vi "Laplacian_kernel.vi"(8 "error in":errorcluster caption="entrée d'erreur", 9 "Y":string[][](array[string]), 10 "X":string[][](array[string]), 11 "laplacian_kernel":cluster{"gamma":string}={"gamma"="None"}) -> (0 "error out":errorcluster caption="sortie d'erreur", 3 "Data":T1)   [LabVIEW 2020]
doc: "Compute the laplacian kernel between X and Y.\n\nThe laplacian kernel is defined as :\n\nK(x, y) = exp(-gamma ||x-y||_1)\n\nfor each pair of rows x in X and y in Y.\n\n\nParameters :\n\n- X : array of shape (n_samples_X, n_features)\n\n- Y : array of shape (n_samples_Y, n_features)\ngammafloat, default None\nIf None, defaults to 1.0 / n_features\n\nReturns : \n\n- kernel_matrix : array of shape (n_samples_X, n_samples_Y)"
uses:
  Laplacian_kernel.lvclass
panel:
  out "Laplacian_kernel.lvclass":refnum<class "Laplacian_kernel.lvclass">
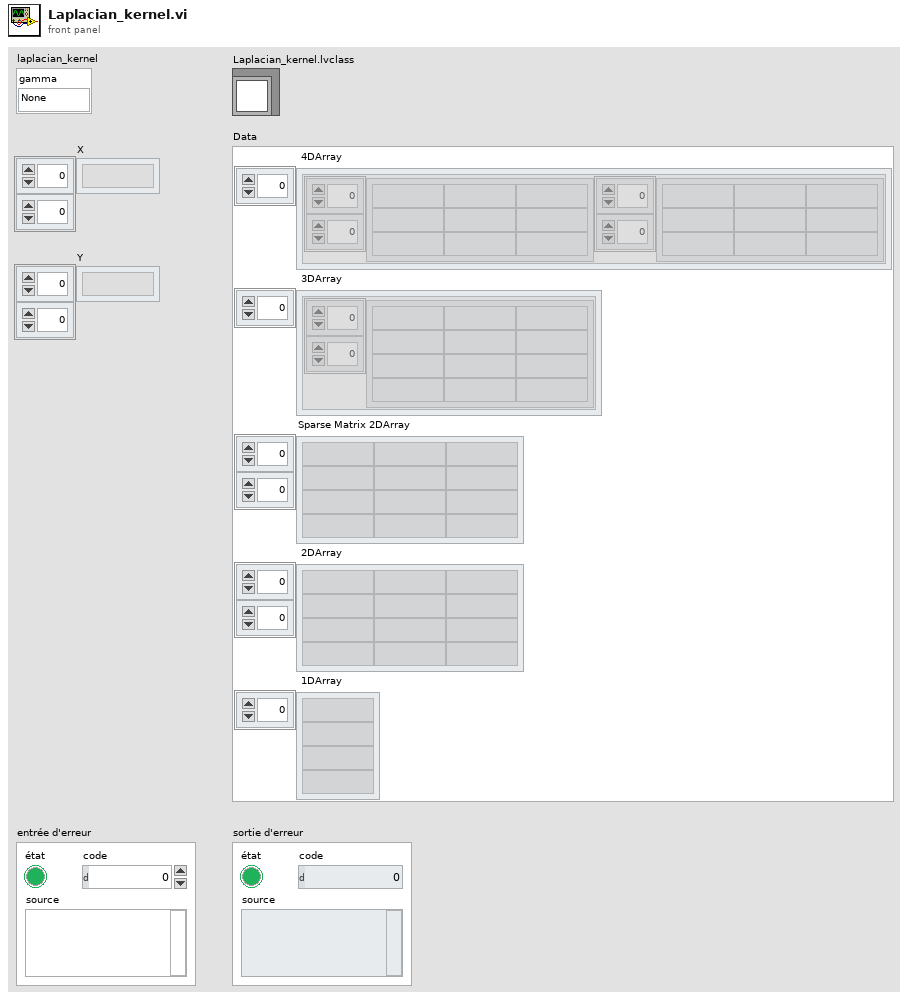
[diagram p1: front panel]
types:
  T1 = cluster{" 4DArray":cluster{"1":string[][], "2":string[][]}[], " 3DArray":cluster{"Tableau":string[][]}[], "Sparse Matrix 2DArray":string[][], " 2DArray":string[][], " 1DArray":string[]}
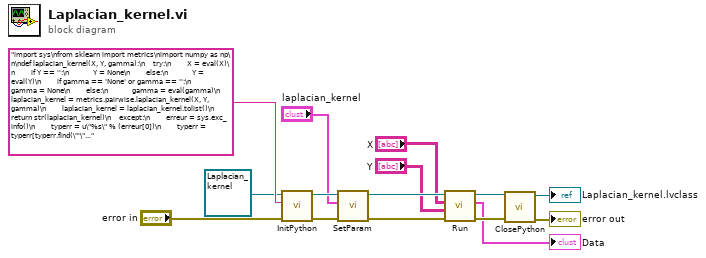
[diagram p0: block diagram]
diagram:
  n1 = call-dynamic "InitPython.vi"("error in (no error)"="error in", "Python Instruction"="import sys\nfrom sklearn import metrics\nimport numpy as np\n\ndef laplacian_kernel(X, Y, gamma):\n    try:\n        X = eval(X)\n        if Y == '':\n            Y = None\n        else:\n            Y = eval(Y)\n        if gamma == 'None' or gamma == '':\n            gamma = None\n        else:\n            gamma = eval(gamma)\n        laplacian_kernel = metrics.pairwise.laplacian_kernel(X, Y, gamma)\n        laplacian_kernel = laplacian_kernel.tolist()\n        return str(laplacian_kernel)\n    except:\n        erreur = sys.exc_info()\n        typerr = u\"%s\" % (erreur[0])\n        typerr = typerr[typerr.find(\"'\")+1:typerr.rfind(\"'\")]\n        msgerr = u\"%s\" % (erreur[1])\n        message = str('/!\\\\ {0} : {1}'. format(typerr,msgerr))\n        return message\n    ", "Scikit-learn en entrée"=refnum<class "Laplacian_kernel.lvclass"> refnum ("Laplacian_kernel.lvclass")) -> ("error out"=w8:errorcluster, "Scikit-learn en sortie"=w11:refnum<class "Laplacian_kernel.lvclass">)  [unwired: 7 in]
  n2 = call-dynamic "SetParam.vi"("error in (no error)"=w8, "laplacian_kernel"="laplacian_kernel", "Laplacian_kernel.lvclass"=w11) -> ("Laplacian_kernel.lvclass"=w9:refnum<class "Laplacian_kernel.lvclass">)  [unwired: 7 in, 1 out]
  n3 = call-dynamic "Run.vi"("error in (no error)"=w8, "Y"="Y", "X"="X", "Laplacian_kernel.lvclass"=w9) -> ("error out"=w6:errorcluster, "Data"=→"Data":T1, "Laplacian_kernel.lvclass"=w7:refnum<class "Laplacian_kernel.lvclass">)  [unwired: 5 in]
  n4 = call-dynamic "ClosePython.vi"("error in (no error)"=w6, "Scikit-learn en entrée"=w7) -> ("error out"=→"error out":errorcluster, "Scikit-learn en sortie"=→"Laplacian_kernel.lvclass":refnum<class "Laplacian_kernel.lvclass">)  [unwired: 8 in]
